vi "Release RProp.vi"(11 "RProp Data":T1) -> ()   [LabVIEW 2015, in "Neural Network.lvclass"]
uses:
  Neural Network.lvclass
  Types/2D Array.ctl
  Types/RProp Algorithm.ctl
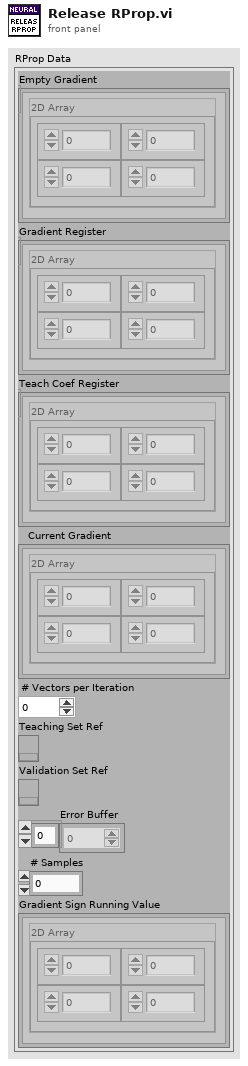
[diagram p1: front panel]
types:
  T1 = typedef "Neural Network.lvclass/RProp Algorithm.ctl" = cluster{"Empty Gradient":T2[], "Gradient Register":T2[], "Teach Coef Register":T2[], "Current Gradient":T2[], "# Vectors per Iteration":i64, "Teaching Set Ref":refnum<k34>, "Validation Set Ref":refnum<k34>, "Error Buffer":dbl[], "# Samples":i64, "Gradient Sign Running Value":T2[]}
  T2 = typedef "Neural Network.lvclass/2D Array.ctl" = cluster{"2D Array":sgl[][]}
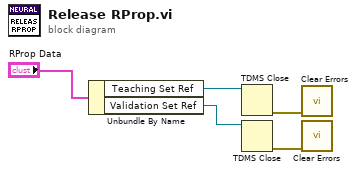
[diagram p0: block diagram]
diagram:
  n1 = Unbundle By Name("RProp Data") -> ("Teaching Set Ref"=w2:refnum<k34>, "Validation Set Ref"=w3:refnum<k34>)
  n2 = TDMS Close(11:w2) -> (0:w4:errorcluster)  [unwired: 1 in, 1 out]
  n3 = TDMS Close(11:w3) -> (0:w5:errorcluster)  [unwired: 1 in, 1 out]
  n4 = call <vilib>:"Clear Errors.vi"("error in (no error)"=w4) -> ()  [unwired: 5 in, 2 out]
  n5 = call <vilib>:"Clear Errors.vi"("error in (no error)"=w5) -> ()  [unwired: 5 in, 2 out]
